vi "Read ParameterNames.vi"(8 "error in (no error)":errorcluster, 11 "ADOParameter in":refnum<class "ADOParameter.lvclass">) -> (0 "error out":errorcluster, 2 "Names":string[](array[string]), 3 "ADOParameter out":refnum<class "ADOParameter.lvclass">)   [LabVIEW 2018]
uses:
  ADOParameter.lvclass
  C:/Viviota/Projects/R&D/LabVIEW_ORM/source/src/Dapper/DynamicParameters/DynamicParameters.lvclass
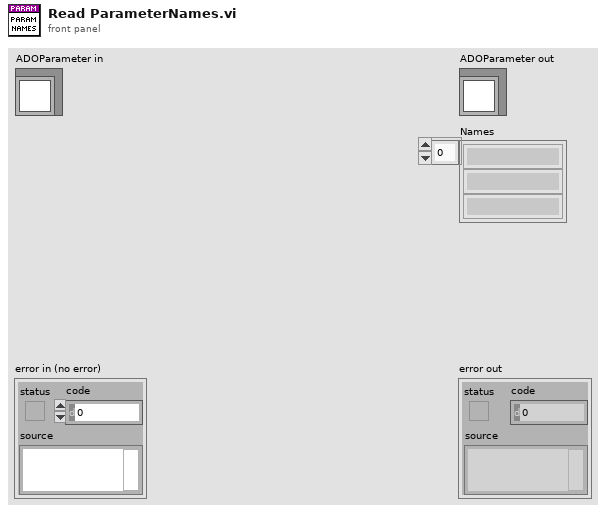
[diagram p1: front panel]
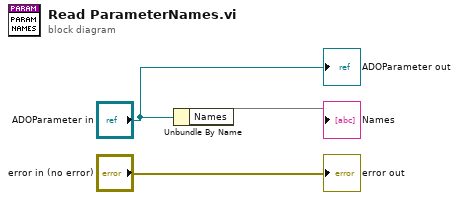
[diagram p0: block diagram]
diagram:
  n1 = Unbundle By Name("ADOParameter in") -> ("Names"=→"Names")
  "error out" <- "error in (no error)"
  "ADOParameter out" <- "ADOParameter in"
